vi "Log_comandos_aquisicion.vi"(8 "Estado":string, 9 "string de Resposta":string, 10 "string de comando":string, 11 "Porta":refnum<visa-resource-name>) -> ()   [LabVIEW 2018]
panel:
  out "Comando":string
  out "before substring":string
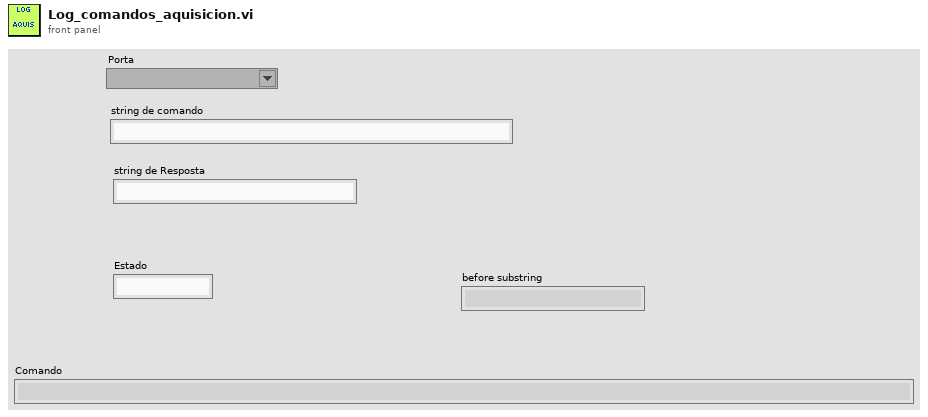
[diagram p1: front panel]
types:
  T1 = enum16{"open", "open or create", "create or replace", "create"}
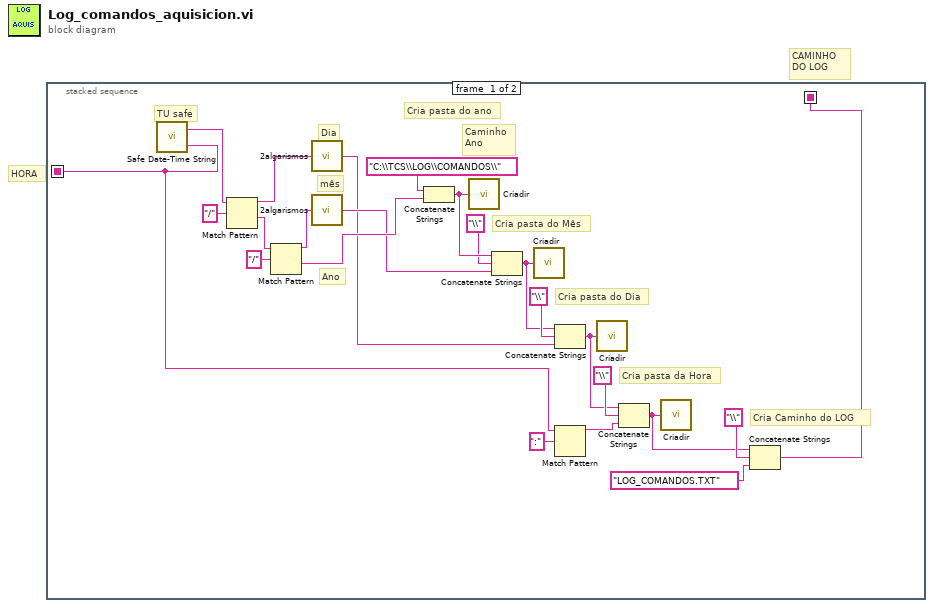
[diagram p0: block diagram]
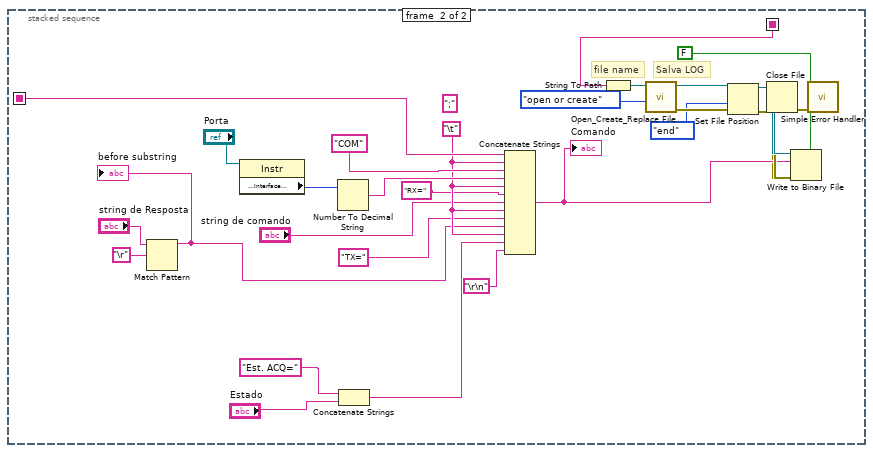
[diagram p2: hidden frame]
diagram:
  # "HORA"
  # "CAMINHO\nDO LOG"
  n1 = stacked-sequence {
    seq-local: [w8 _] -> [_ w38]
    seq-local: [w1 _] -> [_ w48]
    frame #0 {
      # "TU safe"
      # "Cria pasta da Hora"
      # "Cria Caminho do LOG"
      # "Cria pasta do Dia"
      # "Cria pasta do Mês"
      # "Caminho\nAno"
      # "Ano"
      # "mês"
      # "Dia"
      # "Cria pasta do ano"
      n2 = call "Safe Date-Time String.vi"() -> ("Safe time string"=w1:string, "Safe date string"=w2:string)  [unwired: 3 in]
      n3 = Match Pattern(string=w2, regular expression="/") -> (before substring=w20:string, after substring=w21:string)  [unwired: 1 in, 2 out]
      n4 = Match Pattern(string=w21, regular expression="/") -> (before substring=w19:string, after substring=w17:string)  [unwired: 1 in, 2 out]
      n5 = call "2algarismos.vi"("entrada"=w20) -> ("saida"=w11:string)
      n6 = call "2algarismos.vi"("entrada"=w19) -> ("saida"=w14:string)
      n7 = Concatenate Strings("C:\\TCS\\LOG\\COMANDOS\\" ("SOMENTE DIRETORIO"), w17) -> (w16:string)
      n8 = call "Criadir.vi"("SOMENTE DIRETORIO"=w16) -> ()  [unwired: 2 out]
      n9 = Concatenate Strings(w16, "\\" ("regular expression"), w14) -> (w12:string)
      n10 = call "Criadir.vi"("SOMENTE DIRETORIO"=w12) -> ()  [unwired: 2 out]
      n11 = Concatenate Strings(w12, "\\" ("regular expression"), w11) -> (w6:string)
      n12 = Match Pattern(string=w1, regular expression=":") -> (before substring=w4:string)  [unwired: 1 in, 3 out]
      n13 = call "Criadir.vi"("SOMENTE DIRETORIO"=w6) -> ()  [unwired: 2 out]
      n14 = Concatenate Strings(w6, "\\" ("regular expression"), w4) -> (w3:string)
      n15 = call "Criadir.vi"("SOMENTE DIRETORIO"=w3) -> ()  [unwired: 2 out]
      n16 = Concatenate Strings(w3, "\\" ("regular expression"), "LOG_COMANDOS.TXT" ("regular expression")) -> (w8:string)
    }
    frame #1 {
      w34 = "\t"
      (unwired) ";"
      # "Salva LOG"
      # "file name"
      n17 = Match Pattern(string="string de Resposta", regular expression="\r") -> (before substring=w26:string)  [unwired: 1 in, 3 out]
      "before substring" <- w26
      n18 = property class="Instr"(reference="Porta") -> ("Interface Information:Interface Number"=w51:u16)  [unwired: 1 in, 2 out]
      n19 = Number To Decimal String(number=w51) -> (decimal integer string=w49:string)  [unwired: 1 in]
      n20 = Concatenate Strings("Est. ACQ=", "Estado") -> (w32:string)
      n21 = Concatenate Strings(w48, w34, "COM", w49, w34, "RX=", "string de comando", w34, "TX=", w26, w34, w32, "\r\n") -> (w39:string)
      "Comando" <- w39
      n22 = String To Path(string=w38) -> (path=w40:path)
      n23 = call <vilib>:"Open_Create_Replace File.vi"("function (open:0)"=T1."open or create", "file path"=w40) -> ("error out"=w43:errorcluster, "refnum"=w46:refnum<file>)  [unwired: 6 in, 2 out]
      n24 = Set File Position(refnum=w46, from (0:start)=enum16{"start", "end", "current"}."end" ("pos mode (0:2)"), error in=w43) -> (refnum out=w37:refnum<file>, error out=w36:errorcluster)  [unwired: 1 in]
      n25 = Write to Binary File(file (use dialog)=w37, data=w39, error in=w36, 5:FALSE ("prepend array or string size? (T)")) -> (refnum out=w45:refnum<file>, error out=w44:errorcluster)  [unwired: 2 in, 1 out]
      n26 = Close File(refnum=w45, error in=w44) -> (error out=w47:errorcluster)  [unwired: 1 out]
      n27 = call <vilib>:"Simple Error Handler.vi"("error in (no error)"=w47) -> ()  [unwired: 4 in, 5 out]
    }
  }
